vi "HolDrvCtrl_New.vi"(9 "thetaProfiledPID_CTRL":T1={"Controller"={"Kp"=0.0, "Ki"=0.0, "Kd"=0.0, "Period"=0.0, "Max_Integral"=1.0, "Min_Integral"=-1.0, "Max_Input"=0.0, "Min_Input"=0.0, "Continuous"=FALSE, "PositionError"=0.0, "VelocityError"=0.0, "PrevError"=0.0, "Total_Integral"=0.0, "PositionTolerance"=0.05, "VelocityTolerance"=9.99e+35, "SetPoint"=0.0, "Kf"=0.0, "Prev_Deriv"=0.0, "Prev_Deriv 2"=0.0, "DerivativeFilter"=FALSE, "Min_Output"=-9.99e+35, "Max_Output"=9.9e+35, "Prev_F_P"=0.0, "Prev_F_P_2"=0.0, "AntiWindupActive"=FALSE, "Measurement"=0.0, "IntegralZone"=9.9e+30}, "Goal"={"Position"=0.0, "Velocity"=0.0}, "Setpoint"={"Position"=0.0, "Velocity"=0.0}, "Constraint"={"MaxVelocity"=0.0, "MaxAcceleration"=0.0}} {"Constraint"."MaxAcceleration" format="%16_6e"; "Constraint"."MaxVelocity" format="%16_6e"; "Setpoint"."Velocity" format="%16_6e"; "Setpoint"."Position" format="%16_6e"; "Goal"."Velocity" format="%16_6e"; "Goal"."Position" format="%16_6e"; "Controller"."IntegralZone" format="%16_6e"; "Controller"."Measurement" format="%16_6e"; "Controller"."Prev_F_P_2" format="%16_6e"; "Controller"."Prev_F_P" format="%16_6e"; "Controller"."Max_Output" format="%16_6e"; "Controller"."Min_Output" format="%16_6e"; "Controller"."Prev_Deriv 2" format="%16_6e"; "Controller"."Prev_Deriv" format="%16_6e"; "Controller"."Kf" format="%16_6e"; "Controller"."SetPoint" format="%16_6e"; "Controller"."VelocityTolerance" format="%16_6e"; "Controller"."PositionTolerance" format="%16_6e"; "Controller"."Total_Integral" format="%16_6e"; "Controller"."PrevError" format="%16_6e"; "Controller"."VelocityError" format="%16_6e"; "Controller"."PositionError" format="%16_6e"; "Controller"."Min_Input" format="%16_6e"; "Controller"."Max_Input" format="%16_6e"; "Controller"."Min_Integral" format="%16_6e"; "Controller"."Max_Integral" format="%16_6e"; "Controller"."Period" format="%16_6e"; "Controller"."Kd" format="%16_6e"; "Controller"."Ki" format="%16_6e"; "Controller"."Kp" format="%16_6e"}, 10 "yPID_CTRL":T2={"Kp"=0.0, "Ki"=0.0, "Kd"=0.0, "Period"=0.0, "Max_Integral"=1.0, "Min_Integral"=-1.0, "Max_Input"=0.0, "Min_Input"=0.0, "Continuous"=FALSE, "PositionError"=0.0, "VelocityError"=0.0, "PrevError"=0.0, "Total_Integral"=0.0, "PositionTolerance"=0.05, "VelocityTolerance"=9.99e+35, "SetPoint"=0.0, "Kf"=0.0, "Prev_Deriv"=0.0, "Prev_Deriv 2"=0.0, "DerivativeFilter"=FALSE, "Min_Output"=-9.99e+35, "Max_Output"=9.9e+35, "Prev_F_P"=0.0, "Prev_F_P_2"=0.0, "AntiWindupActive"=FALSE, "Measurement"=0.0, "IntegralZone"=9.9e+30} {"IntegralZone" format="%16_6e"; "Measurement" format="%16_6e"; "Prev_F_P_2" format="%16_6e"; "Prev_F_P" format="%16_6e"; "Max_Output" format="%16_6e"; "Min_Output" format="%16_6e"; "Prev_Deriv 2" format="%16_6e"; "Prev_Deriv" format="%16_6e"; "Kf" format="%16_6e"; "SetPoint" format="%16_6e"; "VelocityTolerance" format="%16_6e"; "PositionTolerance" format="%16_6e"; "Total_Integral" format="%16_6e"; "PrevError" format="%16_6e"; "VelocityError" format="%16_6e"; "PositionError" format="%16_6e"; "Min_Input" format="%16_6e"; "Max_Input" format="%16_6e"; "Min_Integral" format="%16_6e"; "Max_Integral" format="%16_6e"; "Period" format="%16_6e"; "Kd" format="%16_6e"; "Ki" format="%16_6e"; "Kp" format="%16_6e"}, 11 "xPID_CTRL":T2={"Kp"=0.0, "Ki"=0.0, "Kd"=0.0, "Period"=0.0, "Max_Integral"=1.0, "Min_Integral"=-1.0, "Max_Input"=0.0, "Min_Input"=0.0, "Continuous"=FALSE, "PositionError"=0.0, "VelocityError"=0.0, "PrevError"=0.0, "Total_Integral"=0.0, "PositionTolerance"=0.05, "VelocityTolerance"=9.99e+35, "SetPoint"=0.0, "Kf"=0.0, "Prev_Deriv"=0.0, "Prev_Deriv 2"=0.0, "DerivativeFilter"=FALSE, "Min_Output"=-9.99e+35, "Max_Output"=9.9e+35, "Prev_F_P"=0.0, "Prev_F_P_2"=0.0, "AntiWindupActive"=FALSE, "Measurement"=0.0, "IntegralZone"=9.9e+30} {"IntegralZone" format="%16_6e"; "Measurement" format="%16_6e"; "Prev_F_P_2" format="%16_6e"; "Prev_F_P" format="%16_6e"; "Max_Output" format="%16_6e"; "Min_Output" format="%16_6e"; "Prev_Deriv 2" format="%16_6e"; "Prev_Deriv" format="%16_6e"; "Kf" format="%16_6e"; "SetPoint" format="%16_6e"; "VelocityTolerance" format="%16_6e"; "PositionTolerance" format="%16_6e"; "Total_Integral" format="%16_6e"; "PrevError" format="%16_6e"; "VelocityError" format="%16_6e"; "PositionError" format="%16_6e"; "Min_Input" format="%16_6e"; "Max_Input" format="%16_6e"; "Min_Integral" format="%16_6e"; "Max_Integral" format="%16_6e"; "Period" format="%16_6e"; "Kd" format="%16_6e"; "Ki" format="%16_6e"; "Kp" format="%16_6e"}) -> (3 "outHOLONOMIC_DRV_CTRL":T5={"poseTolerance"={"TRANSLATION"={"X"=0.0, "Y"=0.0}, "ROTATION"={"VALUE"=0.0, "COS"=1.0, "SIN"=0.0}}, "poseError"={"TRANSLATION"={"X"=0.0, "Y"=0.0}, "ROTATION"={"VALUE"=0.0, "COS"=1.0, "SIN"=0.0}}, "Enabled"=TRUE, "PID_xCtrl"={"Kp"=0.0, "Ki"=0.0, "Kd"=0.0, "Period"=0.0, "Max_Integral"=1.0, "Min_Integral"=-1.0, "Max_Input"=0.0, "Min_Input"=0.0, "Continuous"=FALSE, "PositionError"=0.0, "VelocityError"=0.0, "PrevError"=0.0, "Total_Integral"=0.0, "PositionTolerance"=0.05, "VelocityTolerance"=9.99e+35, "SetPoint"=0.0, "Kf"=0.0, "Prev_Deriv"=0.0, "Prev_Deriv 2"=0.0, "DerivativeFilter"=FALSE, "Min_Output"=-9.99e+35, "Max_Output"=9.9e+35, "Prev_F_P"=0.0, "Prev_F_P_2"=0.0, "AntiWindupActive"=FALSE, "Measurement"=0.0, "IntegralZone"=9.9e+30}, "PID_yCtrl"={"Kp"=0.0, "Ki"=0.0, "Kd"=0.0, "Period"=0.0, "Max_Integral"=1.0, "Min_Integral"=-1.0, "Max_Input"=0.0, "Min_Input"=0.0, "Continuous"=FALSE, "PositionError"=0.0, "VelocityError"=0.0, "PrevError"=0.0, "Total_Integral"=0.0, "PositionTolerance"=0.05, "VelocityTolerance"=9.99e+35, "SetPoint"=0.0, "Kf"=0.0, "Prev_Deriv"=0.0, "Prev_Deriv 2"=0.0, "DerivativeFilter"=FALSE, "Min_Output"=-9.99e+35, "Max_Output"=9.9e+35, "Prev_F_P"=0.0, "Prev_F_P_2"=0.0, "AntiWindupActive"=FALSE, "Measurement"=0.0, "IntegralZone"=9.9e+30}, "PROF_PID_thetaCtrl"={"Controller"={"Kp"=0.0, "Ki"=0.0, "Kd"=0.0, "Period"=0.0, "Max_Integral"=1.0, "Min_Integral"=-1.0, "Max_Input"=0.0, "Min_Input"=0.0, "Continuous"=FALSE, "PositionError"=0.0, "VelocityError"=0.0, "PrevError"=0.0, "Total_Integral"=0.0, "PositionTolerance"=0.05, "VelocityTolerance"=9.99e+35, "SetPoint"=0.0, "Kf"=0.0, "Prev_Deriv"=0.0, "Prev_Deriv 2"=0.0, "DerivativeFilter"=FALSE, "Min_Output"=-9.99e+35, "Max_Output"=9.9e+35, "Prev_F_P"=0.0, "Prev_F_P_2"=0.0, "AntiWindupActive"=FALSE, "Measurement"=0.0, "IntegralZone"=9.9e+30}, "Goal"={"Position"=0.0, "Velocity"=0.0}, "Setpoint"={"Position"=0.0, "Velocity"=0.0}, "Constraint"={"MaxVelocity"=0.0, "MaxAcceleration"=0.0}}, "RotationError"={"VALUE"=0.0, "COS"=1.0, "SIN"=0.0}, "FirstRun"=FALSE} {"RotationError"."SIN" format="%13.4f"; "RotationError"."COS" format="%13.4f"; "RotationError"."VALUE" format="%13.4f"; "PROF_PID_thetaCtrl"."Constraint"."MaxAcceleration" format="%16_6e"; "PROF_PID_thetaCtrl"."Constraint"."MaxVelocity" format="%16_6e"; "PROF_PID_thetaCtrl"."Setpoint"."Velocity" format="%16_6e"; "PROF_PID_thetaCtrl"."Setpoint"."Position" format="%16_6e"; "PROF_PID_thetaCtrl"."Goal"."Velocity" format="%16_6e"; "PROF_PID_thetaCtrl"."Goal"."Position" format="%16_6e"; "PROF_PID_thetaCtrl"."Controller"."IntegralZone" format="%16_6e"; "PROF_PID_thetaCtrl"."Controller"."Measurement" format="%16_6e"; "PROF_PID_thetaCtrl"."Controller"."Prev_F_P_2" format="%16_6e"; "PROF_PID_thetaCtrl"."Controller"."Prev_F_P" format="%16_6e"; "PROF_PID_thetaCtrl"."Controller"."Max_Output" format="%16_6e"; "PROF_PID_thetaCtrl"."Controller"."Min_Output" format="%16_6e"; "PROF_PID_thetaCtrl"."Controller"."Prev_Deriv 2" format="%16_6e"; "PROF_PID_thetaCtrl"."Controller"."Prev_Deriv" format="%16_6e"; "PROF_PID_thetaCtrl"."Controller"."Kf" format="%16_6e"; "PROF_PID_thetaCtrl"."Controller"."SetPoint" format="%16_6e"; "PROF_PID_thetaCtrl"."Controller"."VelocityTolerance" format="%16_6e"; "PROF_PID_thetaCtrl"."Controller"."PositionTolerance" format="%16_6e"; "PROF_PID_thetaCtrl"."Controller"."Total_Integral" format="%16_6e"; "PROF_PID_thetaCtrl"."Controller"."PrevError" format="%16_6e"; "PROF_PID_thetaCtrl"."Controller"."VelocityError" format="%16_6e"; "PROF_PID_thetaCtrl"."Controller"."PositionError" format="%16_6e"; "PROF_PID_thetaCtrl"."Controller"."Min_Input" format="%16_6e"; "PROF_PID_thetaCtrl"."Controller"."Max_Input" format="%16_6e"; "PROF_PID_thetaCtrl"."Controller"."Min_Integral" format="%16_6e"; "PROF_PID_thetaCtrl"."Controller"."Max_Integral" format="%16_6e"; "PROF_PID_thetaCtrl"."Controller"."Period" format="%16_6e"; "PROF_PID_thetaCtrl"."Controller"."Kd" format="%16_6e"; "PROF_PID_thetaCtrl"."Controller"."Ki" format="%16_6e"; "PROF_PID_thetaCtrl"."Controller"."Kp" format="%16_6e"; "PID_yCtrl"."IntegralZone" format="%16_6e"; "PID_yCtrl"."Measurement" format="%16_6e"; "PID_yCtrl"."Prev_F_P_2" format="%16_6e"; "PID_yCtrl"."Prev_F_P" format="%16_6e"; "PID_yCtrl"."Max_Output" format="%16_6e"; "PID_yCtrl"."Min_Output" format="%16_6e"; "PID_yCtrl"."Prev_Deriv 2" format="%16_6e"; "PID_yCtrl"."Prev_Deriv" format="%16_6e"; "PID_yCtrl"."Kf" format="%16_6e"; "PID_yCtrl"."SetPoint" format="%16_6e"; "PID_yCtrl"."VelocityTolerance" format="%16_6e"; "PID_yCtrl"."PositionTolerance" format="%16_6e"; "PID_yCtrl"."Total_Integral" format="%16_6e"; "PID_yCtrl"."PrevError" format="%16_6e"; "PID_yCtrl"."VelocityError" format="%16_6e"; "PID_yCtrl"."PositionError" format="%16_6e"; "PID_yCtrl"."Min_Input" format="%16_6e"; "PID_yCtrl"."Max_Input" format="%16_6e"; "PID_yCtrl"."Min_Integral" format="%16_6e"; "PID_yCtrl"."Max_Integral" format="%16_6e"; "PID_yCtrl"."Period" format="%16_6e"; "PID_yCtrl"."Kd" format="%16_6e"; "PID_yCtrl"."Ki" format="%16_6e"; "PID_yCtrl"."Kp" format="%16_6e"; "PID_xCtrl"."IntegralZone" format="%16_6e"; "PID_xCtrl"."Measurement" format="%16_6e"; "PID_xCtrl"."Prev_F_P_2" format="%16_6e"; "PID_xCtrl"."Prev_F_P" format="%16_6e"; "PID_xCtrl"."Max_Output" format="%16_6e"; "PID_xCtrl"."Min_Output" format="%16_6e"; "PID_xCtrl"."Prev_Deriv 2" format="%16_6e"; "PID_xCtrl"."Prev_Deriv" format="%16_6e"; "PID_xCtrl"."Kf" format="%16_6e"; "PID_xCtrl"."SetPoint" format="%16_6e"; "PID_xCtrl"."VelocityTolerance" format="%16_6e"; "PID_xCtrl"."PositionTolerance" format="%16_6e"; "PID_xCtrl"."Total_Integral" format="%16_6e"; "PID_xCtrl"."PrevError" format="%16_6e"; "PID_xCtrl"."VelocityError" format="%16_6e"; "PID_xCtrl"."PositionError" format="%16_6e"; "PID_xCtrl"."Min_Input" format="%16_6e"; "PID_xCtrl"."Max_Input" format="%16_6e"; "PID_xCtrl"."Min_Integral" format="%16_6e"; "PID_xCtrl"."Max_Integral" format="%16_6e"; "PID_xCtrl"."Period" format="%16_6e"; "PID_xCtrl"."Kd" format="%16_6e"; "PID_xCtrl"."Ki" format="%16_6e"; "PID_xCtrl"."Kp" format="%16_6e"; "poseError"."ROTATION"."SIN" format="%13.4f"; "poseError"."ROTATION"."COS" format="%13.4f"; "poseError"."ROTATION"."VALUE" format="%13.4f"; "poseError"."TRANSLATION"."Y" format="%14.3f"; "poseError"."TRANSLATION"."X" format="%14.3f"; "poseTolerance"."ROTATION"."SIN" format="%13.4f"; "poseTolerance"."ROTATION"."COS" format="%13.4f"; "poseTolerance"."ROTATION"."VALUE" format="%13.4f"; "poseTolerance"."TRANSLATION"."Y" format="%14.3f"; "poseTolerance"."TRANSLATION"."X" format="%14.3f"})   [LabVIEW 2019, in "Trajectory_Library.lvlib"]
doc: "This holonomic drive controller can be used to follow trajectories using a holonomic drivetrain (i.e. swerve or mecanum). Holonomic trajectory following is a much simpler problem to solve compared to skid-steer style drivetrains because it is possible to individually control forward, sideways, and angular velocity.\n\nThe holonomic drive controller takes in one PID controller for each direction, forward and sideways, and one profiled PID controller for the angular direction. Because the heading dynamics are decoupled from translations, users can specify a custom heading that the drivetrain should point toward. This heading reference is profiled for smoothness.\n\nThis VI constructs a holonomic drive controller data structure.\n \nInputs:\n - xController -- A PID Controller to respond to error in the field-relative x direction.\n - yController -- A PID Controller to respond to error in the field-relative y direction.\n - thetaController -- A profiled PID controller to respond to error in angle.\n\nOutput:\n - outHolonomicDrvCtrl -- controller data structure."
uses:
  Trajectory_Library.lvlib
  TypeDef/HOLONOMIC_DRV_CTRL.ctl
  TypeDef/POSE2D.ctl
  TypeDef/TRANSLATION2D.ctl
  TypeDef/ROTATION2D.ctl
  TypeDef/PID_CONTROLLER.ctl
  TypeDef/PROFILED_PID_CONTROLLER.ctl
  TypeDef/TRAPEZOID_PROFILE_STATE.ctl
  TypeDef/TRAPEZOID_PROFILE_CONSTRAINT.ctl
  PIDController_EnableContinousInput.vi
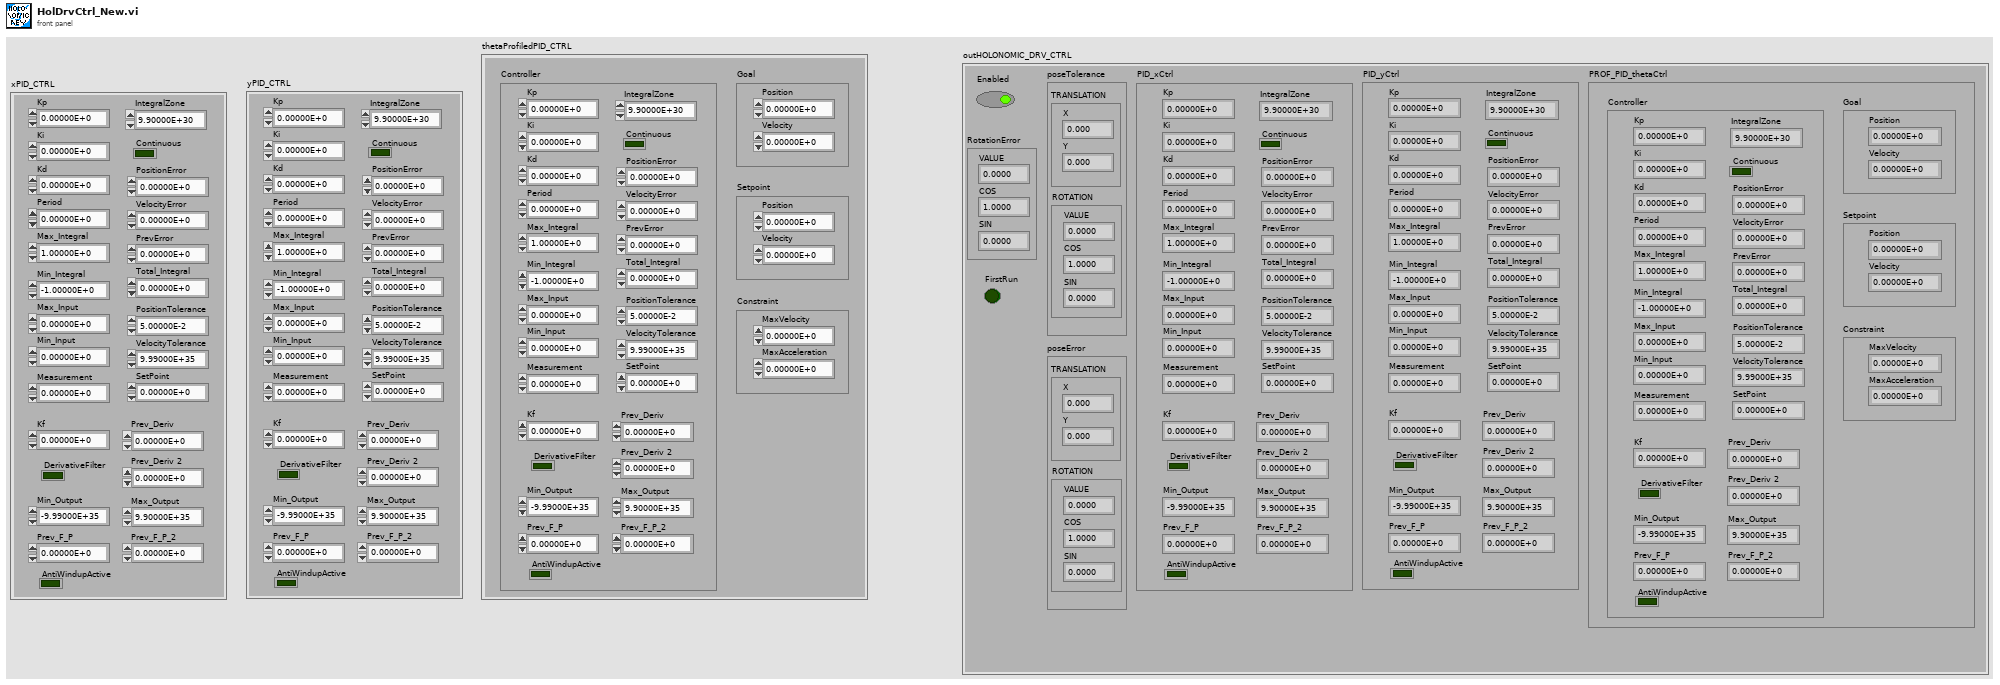
[diagram p1: front panel]
types:
  T1 = typedef "Trajectory_Library.lvlib/PROFILED_PID_CONTROLLER.ctl" = cluster{"Controller":T2, "Goal":T3, "Setpoint":T3, "Constraint":T4}
  T2 = typedef "Trajectory_Library.lvlib/PID_CONTROLLER.ctl" = cluster{"Kp":dbl, "Ki":dbl, "Kd":dbl, "Period":dbl, "Max_Integral":dbl, "Min_Integral":dbl, "Max_Input":dbl, "Min_Input":dbl, "Continuous":bool, "PositionError":dbl, "VelocityError":dbl, "PrevError":dbl, "Total_Integral":dbl, "PositionTolerance":dbl, "VelocityTolerance":dbl, "SetPoint":dbl, "Kf":dbl, "Prev_Deriv":dbl, "Prev_Deriv 2":dbl, "DerivativeFilter":bool, "Min_Output":dbl, "Max_Output":dbl, "Prev_F_P":dbl, "Prev_F_P_2":dbl, "AntiWindupActive":bool, "Measurement":dbl, "IntegralZone":dbl}
  T3 = typedef "Trajectory_Library.lvlib/TRAPEZOID_PROFILE_STATE.ctl" = cluster{"Position":dbl, "Velocity":dbl}
  T4 = typedef "Trajectory_Library.lvlib/TRAPEZOID_PROFILE_CONSTRAINT.ctl" = cluster{"MaxVelocity":dbl, "MaxAcceleration":dbl}
  T5 = typedef "Trajectory_Library.lvlib/HOLONOMIC_DRV_CTRL.ctl" = cluster{"poseTolerance":T6, "poseError":T6, "Enabled":bool, "PID_xCtrl":T2, "PID_yCtrl":T2, "PROF_PID_thetaCtrl":T1, "RotationError":T8, "FirstRun":bool}
  T6 = typedef "Trajectory_Library.lvlib/POSE2D.ctl" = cluster{"TRANSLATION":T7, "ROTATION":T8}
  T7 = typedef "Trajectory_Library.lvlib/TRANSLATION2D.ctl" = cluster{"X":dbl, "Y":dbl}
  T8 = typedef "Trajectory_Library.lvlib/ROTATION2D.ctl" = cluster{"VALUE":dbl, "COS":dbl, "SIN":dbl}
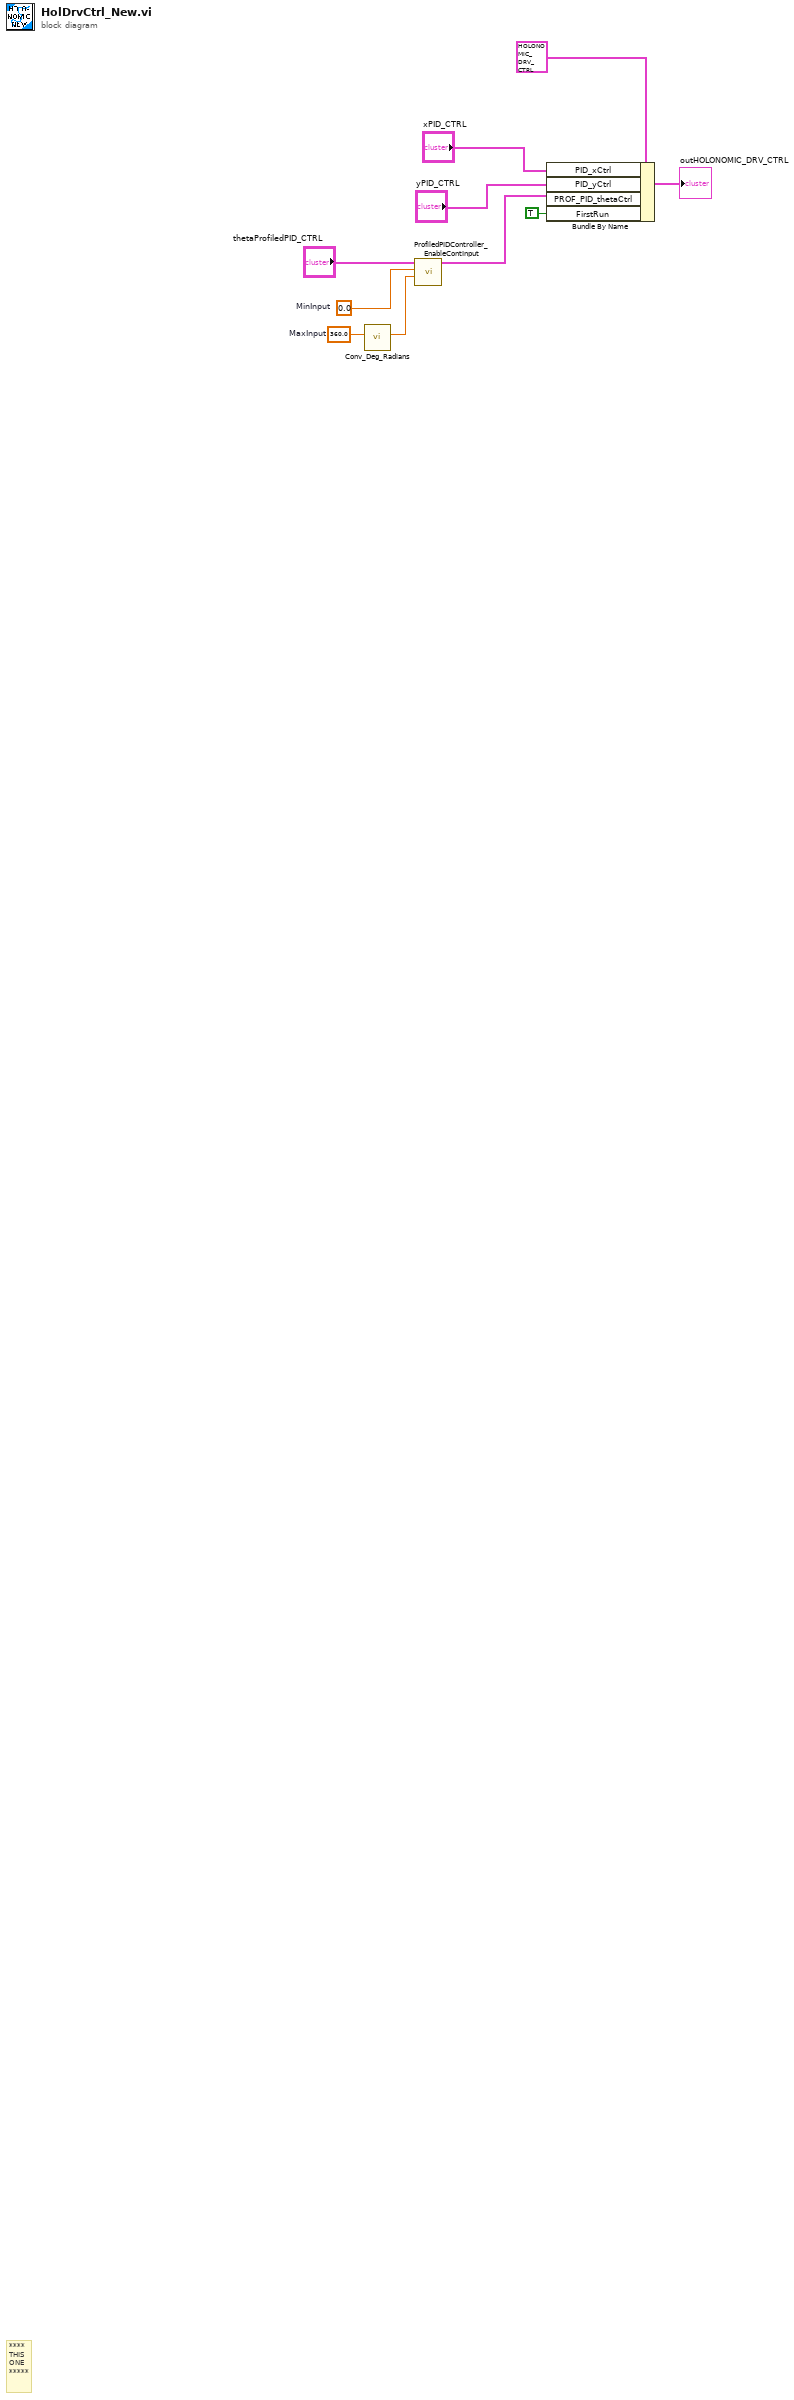
[diagram p0: block diagram]
diagram:
  w3 = 0.0  # MinInput
  w2 = 360.0  # MaxInput
  # "****\nTHIS\nONE\n*****"
  n1 = call "Conv_Deg_Radians.vi"("Degress"=w2) -> ("Radians"=w1:dbl)  [unwired: 10 in]
  n2 = call "ProfiledPIDController_EnableContInput.vi"("MaxInput"=w1, "MinInput"=w3, "in PROFILED_PID_CONTROLLER"="thetaProfiledPID_CTRL") -> ("out PROFILED_PID_CONTROLLER"=w4:T1)  [unwired: 8 in]
  n3 = Bundle By Name(cluster=T5 {"poseTolerance"={"TRANSLATION"={"X"=0.0, "Y"=0.0}, "ROTATION"={"VALUE"=0.0, "COS"=1.0, "SIN"=0.0}}, "poseError"={"TRANSLATION"={"X"=0.0, "Y"=0.0}, "ROTATION"={"VALUE"=0.0, "COS"=1.0, "SIN"=0.0}}, "Enabled"=TRUE, "PID_xCtrl"={"Kp"=0.0, "Ki"=0.0, "Kd"=0.0, "Period"=0.0, "Max_Integral"=1.0, "Min_Integral"=-1.0, "Max_Input"=0.0, "Min_Input"=0.0, "Continuous"=FALSE, "PositionError"=0.0, "VelocityError"=0.0, "PrevError"=0.0, "Total_Integral"=0.0, "PositionTolerance"=0.05, "VelocityTolerance"=9.99e+35, "SetPoint"=0.0, "Kf"=0.0, "Prev_Deriv"=0.0, "Prev_Deriv 2"=0.0, "DerivativeFilter"=FALSE, "Min_Output"=-9.99e+35, "Max_Output"=9.9e+35, "Prev_F_P"=0.0, "Prev_F_P_2"=0.0, "AntiWindupActive"=FALSE, "Measurement"=0.0, "IntegralZone"=9.9e+30}, "PID_yCtrl"={"Kp"=0.0, "Ki"=0.0, "Kd"=0.0, "Period"=0.0, "Max_Integral"=1.0, "Min_Integral"=-1.0, "Max_Input"=0.0, "Min_Input"=0.0, "Continuous"=FALSE, "PositionError"=0.0, "VelocityError"=0.0, "PrevError"=0.0, "Total_Integral"=0.0, "PositionTolerance"=0.05, "VelocityTolerance"=9.99e+35, "SetPoint"=0.0, "Kf"=0.0, "Prev_Deriv"=0.0, "Prev_Deriv 2"=0.0, "DerivativeFilter"=FALSE, "Min_Output"=-9.99e+35, "Max_Output"=9.9e+35, "Prev_F_P"=0.0, "Prev_F_P_2"=0.0, "AntiWindupActive"=FALSE, "Measurement"=0.0, "IntegralZone"=9.9e+30}, "PROF_PID_thetaCtrl"={"Controller"={"Kp"=0.0, "Ki"=0.0, "Kd"=0.0, "Period"=0.0, "Max_Integral"=1.0, "Min_Integral"=-1.0, "Max_Input"=0.0, "Min_Input"=0.0, "Continuous"=FALSE, "PositionError"=0.0, "VelocityError"=0.0, "PrevError"=0.0, "Total_Integral"=0.0, "PositionTolerance"=0.05, "VelocityTolerance"=9.99e+35, "SetPoint"=0.0, "Kf"=0.0, "Prev_Deriv"=0.0, "Prev_Deriv 2"=0.0, "DerivativeFilter"=FALSE, "Min_Output"=-9.99e+35, "Max_Output"=9.9e+35, "Prev_F_P"=0.0, "Prev_F_P_2"=0.0, "AntiWindupActive"=FALSE, "Measurement"=0.0, "IntegralZone"=9.9e+30}, "Goal"={"Position"=0.0, "Velocity"=0.0}, "Setpoint"={"Position"=0.0, "Velocity"=0.0}, "Constraint"={"MaxVelocity"=0.0, "MaxAcceleration"=0.0}}, "RotationError"={"VALUE"=0.0, "COS"=1.0, "SIN"=0.0}, "FirstRun"=FALSE} ("HOLONOMIC_DRV_CTRL"), "PID_xCtrl"="xPID_CTRL", "PID_yCtrl"="yPID_CTRL", "PROF_PID_thetaCtrl"=w4, "FirstRun"=TRUE) -> (→"outHOLONOMIC_DRV_CTRL":T5)
